vi "solar_excel Create.vi"(6 "Visible? (F)":bool, 7 "Worksheet":string, 8 "error in (no error)":errorcluster, 10 "Cells":string[][](array[string]), 11 "Excel Workbook (*.xlsx)":path) -> (0 "error out":errorcluster, 3 "dup Excel Workbook":path)   [LabVIEW 2018]
doc: "This creates an Excel workbook."
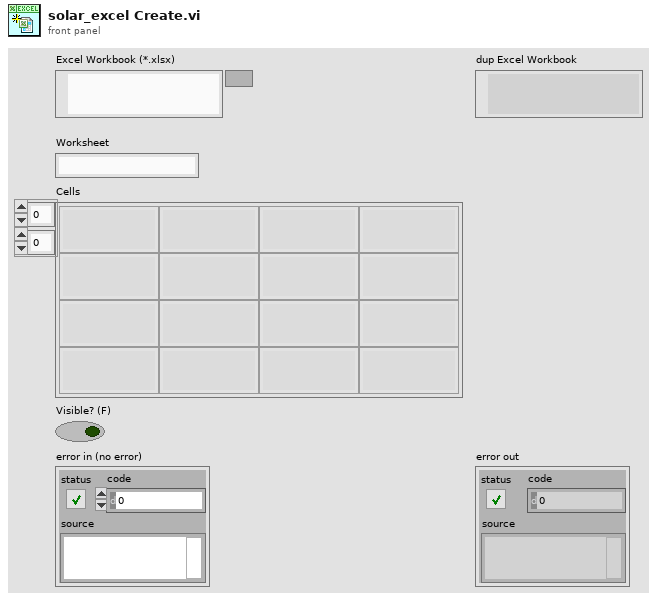
[diagram p1: front panel]
types:
  T1 = typedef "solar_excel_ctl App.ctl" = cluster{"ExcelApp":refnum<k7>, "Workbooks":refnum<k7>, "TSV":refnum<queue>}
  T2 = typedef "solar_excel_ctl Workbook.ctl" = cluster{"ExcelApp":refnum<k7>, "Workbooks":refnum<k7>, "TSV":refnum<queue>, "OpenWkb":refnum<k7>}
  T3 = typedef "solar_excel_ctl Worksheet.ctl" = cluster{"ExcelApp":refnum<k7>, "Workbooks":refnum<k7>, "TSV":refnum<queue>, "OpenWkb":refnum<k7>, "Worksheets":refnum<k7>, "OpenWksh":refnum<k7>}
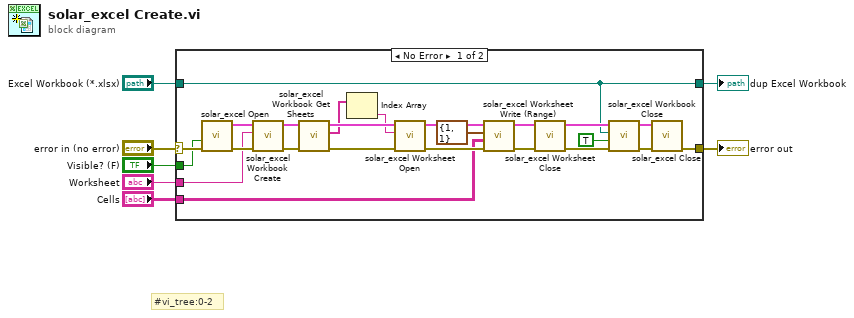
[diagram p0: block diagram]
diagram:
  # "#vi_tree:0-2"
  n1 = case shown="No Error" "error in (no error)" {
    selector: "error in (no error)" -> [w31 w33]
    tunnel: [w30 w33] -> w6
    tunnel: "Worksheet" -> [w20 _]
    tunnel: "Excel Workbook (*.xlsx)" -> [w8 w32]
    tunnel: "Cells" -> [w11 _]
    tunnel: "Visible? (F)" -> [w9 _]
    tunnel: [w8 w32] -> w1
    frame No Error {
      n2 = call "solar_excel Open.vi"("error in (no error)"=w31, "Visible? (F)"=w9) -> ("error out"=w29:errorcluster, "Excel App"=w28:T1)  [unwired: 8 in]
      n3 = call "solar_excel Workbook Create.vi"("error in (no error)"=w29, "Worksheet"=w20, "Excel App"=w28) -> ("error out"=w24:errorcluster, "Excel Workbook"=w22:T2)  [unwired: 7 in]
      n4 = call "solar_excel Workbook Get Sheets.vi"("error in (no error)"=w24, "Excel Workbook in"=w22) -> ("error out"=w23:errorcluster, "Worksheet Names"=w19:string[], "Excel Workbook out"=w21:T2)  [unwired: 6 in, 1 out]
      n5 = Index Array(array=w19) -> (element=w18:string)  [unwired: 1 in]
      n6 = call "solar_excel Worksheet Open.vi"("error in (no error)"=w23, "Sheet Name (STR) or Number (I32)"=w18, "Excel Workbook"=w21) -> ("error out"=w25:errorcluster, "Excel Worksheet"=w17:T3)  [unwired: 5 in, 2 out]
      n7 = call "solar_excel Worksheet Write (Range).vi"("error in (no error)"=w25, "Cells"=w11, "Start (1,1 = 'A1')"=cluster{"Row":u32, "Column":u32} {"Row"=1, "Column"=1}, "Excel Worksheet in"=w17) -> ("error out"=w26:errorcluster, "Excel Worksheet out"=w16:T3)  [unwired: 6 in]
      n8 = call "solar_excel Worksheet Close.vi"("error in (no error)"=w26, "Excel Worksheet"=w16) -> ("error out"=w15:errorcluster, "Excel Workbook"=w14:T2)  [unwired: 8 in]
      n9 = call "solar_excel Workbook Close.vi"("error in (no error)"=w15, "Save? (F)"=TRUE, "Excel Workbook (*.xlsx)"=w8, "Excel Workbook"=w14) -> ("error out"=w27:errorcluster, "Excel App"=w13:T1)  [unwired: 6 in]
      n10 = call "solar_excel Close.vi"("error in (no error)"=w27, "Excel App"=w13) -> ("error out"=w30:errorcluster)  [unwired: 9 in]
    }
    frame Error {
    }
  }
  "error out" <- w6
  "dup Excel Workbook" <- w1
